vi "Read Grid Colors.vi"(9 "GraphScale in":refnum<class "GraphScale.lvclass">) -> (3 "GraphScale out":refnum<class "GraphScale.lvclass">, 4 "Grid Colors":cluster{"Major Color":u32, "Minor Color":u32})   [LabVIEW 2014, in "GraphScale.lvclass"]
uses:
  GraphScale.lvclass
  GraphScale.lvclass/GraphScale.ctl
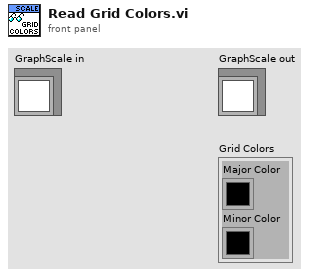
[diagram p1: front panel]
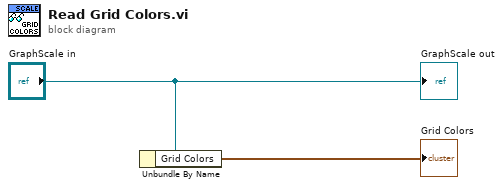
[diagram p0: block diagram]
diagram:
  n1 = Unbundle By Name("GraphScale in") -> ("Grid Colors"=→"Grid Colors":cluster{"Major Color":u32, "Minor Color":u32})
  "GraphScale out" <- "GraphScale in"
